vi "Close.vi"(8 "error in":errorcluster, 11 "Editor Control Base in":refnum<class "Editor Control Base.lvclass">) -> (0 "error out":errorcluster, 3 "Editor Control Base out":refnum<class "Editor Control Base.lvclass">)   [LabVIEW 2024, in "SourceGrid.lvlib" / "Editor Control Base.lvclass"]
uses:
  Editor Control Base.lvclass
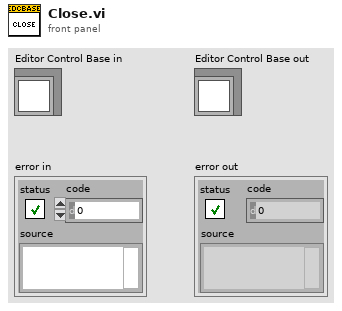
[diagram p1: front panel]
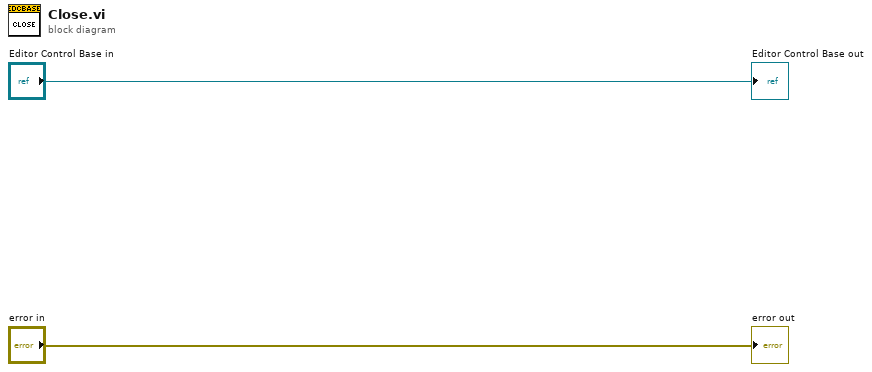
[diagram p0: block diagram]
diagram:
  "error out" <- "error in"
  "Editor Control Base out" <- "Editor Control Base in"
